vi "Write json to AIParam one test.vi"(10 "JSON Data In":string="AI  SET\n {\"GM1QN3_XQ01\":{\"instrument_gain\":10,\n                                    \"input_register_min\":6554,\n                                     \"input_register_max\":32767,\n                                     \"input_pv_max\":2.5},\n \"GM1QN4_XQ01\":{\"instrument_gain\":10,\n                                    \"input_register_min\":6554,\n                                     \"input_register_max\":32767,\n                                      \"input_pv_max\":4.99}\n}") -> (0 "error out":errorcluster)   [LabVIEW 2019]
uses:
  Database/ctl/Coninfo.ctl
  projects/Additivs/Regulators/PROG/GM1_201007/enums/KFM.ctl
  projects/Additivs/Regulators/PROG/GM1_201007/enums/AI.ctl
  projects/Graphetron_1/Heater/PROG/GM3_200601/enums/AI.ctl
  projects/Graphetron_1/Heater/PROG/GM3_200601/enums/KFM.ctl
  Transform/JSON to array.vi
  <vilib>/JDP Science/JSONtext/Find Multiple Items.vi
  <vilib>/JDP Science/JSONtext/String Subset.vi
  <vilib>/JDP Science/JSONtext/support/Strip Quotes and Unescape.vi
  <vilib>/JDP Science/JSONtext/Parsing/Parse Full Path or Item Name.vi
  <vilib>/JDP Science/JSONtext/Offset/Find Item Locations by Path.vi
  <vilib>/JDP Science/JSONtext/support/Unescape JSON string.vi
  <vilib>/JDP Science/JSONtext/Get Array Elements.vi
  projects/Graphetron_1/Heater/PROG/GM3_200601/enums/Param_gm3.lvlib
  Inputs.lvlib
  Database/PostgreSQL.lvlib
  projects/Additivs/Regulators/PROG/GM1_201007/enums/Param_h0gm1.lvlib
panel:
  in  "Set":bool
  in  "password":string
  in  "stop":bool
  out "data value 3":dbl[][](array[numeric])
  out "Names":string[][](array[string])
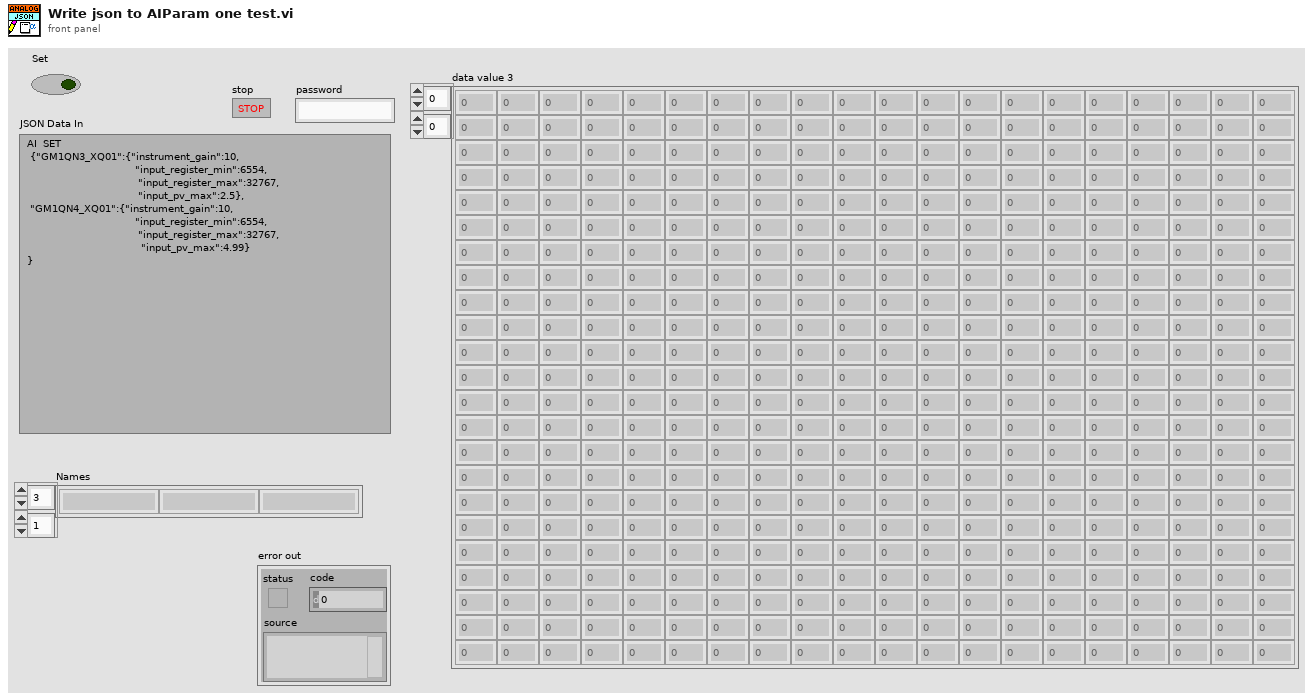
[diagram p1: front panel]
types:
  T1 = typedef "Param_h0gm1.lvlib/AI.ctl" = enum16{"GM1QN1_XQ01", "GM1QN2_XQ01", "GM1QN3_XQ01", "GM1QN4_XQ01", "GM1QN5_XQ01", "GM1QN6_XQ01", "GM1QN7_XQ01", "GM1QN8_XQ01", "GM1QN9_XQ01", "GM1QN10_XQ01", "GM1QN11_XQ01", "GM1QN12_XQ01", "GM1QN13_XQ01", "GM1QN14_XQ01", "GM1QN15_XQ01", "GM1QN16_XQ01", "GM1QN17_XQ01", "GM1QN18_XQ01", "GM1QN19_XQ01", "GM1QN20_XQ01", "GM1QN21_XQ01", "GM1QN22_XQ01", "GM1QN23_XQ01"}
  T2 = typedef "Param_h0gm1.lvlib/KFM.ctl" = enum16{"GM1JBA1_JA1", "GM1JBA1_JA2", "GM1JBA2_JA1", "GM1JBA2_JA2", "GM1JBA3_JA1"}
  T3 = typedef "PostgreSQL.lvlib/Coninfo.ctl" = cluster{"host":string, "port":string, "client_encoding":string, "dbname":string, "user":string, "password":string}
  T4 = enum16{"GM3KF1_A1", "EB2TB1_2TB1", "EB2TB2_2TB2", "EB2TB3_2TB3", "EB2TF1_A13", "EB2TF1_A131", "EB3TB1_3TB1", "EB3TB2_3TB2", "EB3TB3_3TB3", "GM2KF1_A1", "GM2KF1_A11", "GM2KF1_A12", "GM2KF1_A14", "GM2KF1_A15", "GM2KF1_A19", "GM2TF3_A117", "GM2TF3_A118", "GM3JBA1_A13", "GM3KF1_A11", "GM3KF1_A12", "GM3KF1_A15", "GM3KF1_A16", "GM3KF1_A17", "GM3KF1_A18", "GM3KF1_A19", "GM3TF1_A111", "GM3TF1_A112", "GM3TF1_A113", "GM3TF1_A114", "GM3TF1_A116", "GM3TF1_A117", "GM3TF1_A118", "GM3TF1_A14", "HXTF1_A11", "HXTF1_A14", "HXTF2_A15", "W2JBA1_A2", "W2JBA2_A2", "W2JBA3_A2", "W2JBA4_A2", "W2JBA5_A1"}
  T5 = typedef "Param_gm3.lvlib/KFM.ctl" = enum16{"GM3.KF1_A1", "EB2.TB.1_2TB1", "EB2.TB.2_2TB2", "EB2.TB.3_2TB3", "EB2.TF1_A13", "EB2.TF1_A131", "EB3.TB.1_3TB1", "EB3.TB.2_3TB2", "EB3.TB.3_3TB3", "GM2.KF1_A1", "GM2.KF1_A11", "GM2.KF1_A12", "GM2.KF1_A14", "GM2.KF1_A15", "GM2.KF1_A19", "GM2.TF3_A117", "GM2.TF3_A118", "GM3.JBA1_A13", "GM3.KF1_A11", "GM3.KF1_A12", "GM3.KF1_A15", "GM3.KF1_A16", "GM3.KF1_A17", "GM3.KF1_A18", "GM3.KF1_A19", "GM3.TF1_A111", "GM3.TF1_A112", "GM3.TF1_A113", "GM3.TF1_A114", "GM3.TF1_A116", "GM3.TF1_A117", "GM3.TF1_A118", "GM3.TF1_A14", "HX.TF1_A11", "HX.TF1_A14", "HX.TF2_A15", "W2.JBA1_A2", "W2.JBA2_A2", "W2.JBA3_A2", "W2.JBA4_A2", "W2.JBA5_A1"}
  T6 = enum16{"EB2BC11", "EB2BC12", "EB2BC21", "EB2BC22", "EB2BP1", "EB2BT1", "EB2BT2", "EB2BT3", "EB2BT4", "EB2BT5", "EB2QN1", "EB2QN2", "EB2TB1_BA1", "EB2TB1_BC1", "EB2TB1_BE1", "EB2TB1_BJ1", "EB2TB2_BA2", "EB2TB2_BC2", "EB2TB2_BE2", "EB2TB2_BJ2", "EB2TB3_BA3", "EB2TB3_BC3", "EB2TB3_BE3", "EB2TB3_BJ3", "EB2TB_BJ", "EB2_BC1", "EB2_BC2", "EB3BP1", "EB3BT11", "EB3BT12", "EB3BT21", "EB3BT22", "EB3BT31", "EB3BT32", "EB3QN1", "EB3QN2", "EB3TB1_BA1", "EB3TB1_BC1", "EB3TB1_BE1", "EB3TB1_BJ1", "EB3TB2_BA2", "EB3TB2_BC2", "EB3TB2_BE2", "EB3TB2_BJ2", "EB3TB3_BA3", "EB3TB3_BC3", "EB3TB3_BE3", "EB3TB3_BJ3", "EB3TB_BJ", "EB3_BC1", "EB3_BC2", "GM2EP1BT1", "GM2EP1BT10", "GM2EP1BT11", "GM2EP1BT2", "GM2EP1BT3", "GM2EP1BT4", "GM2EP1BT5", "GM2EP1BT6", "GM2EP1BT7", "GM2EP1BT8", "GM2EP1BT9", "GM31BP1", "GM31BP2", "GM31BW1", "GM31BW1_BQ01", "GM31BW1_BQ03", "GM31BW1_XZ01", "GM31BW2", "GM31BW2_BQ01", "GM31BW2_XZ01", "GM31QN1", "GM32BP1", "GM32QN1", "GM32QN2", "GM3HT1BC1", "GM3HT1BC2", "GM3HT1BT1", "GM3HT1BT2", "HW3BT1", "HW3BT2", "HW3BT3"}
  T7 = typedef "Param_gm3.lvlib/AI.ctl" = enum16{"EB2.BC11", "EB2.BC12", "EB2.BC21", "EB2.BC22", "EB2.BP1", "EB2.BT1", "EB2.BT2", "EB2.BT3", "EB2.BT4", "EB2.BT5", "EB2.QN1", "EB2.QN2", "EB2.TB.1_BA1", "EB2.TB.1_BC1", "EB2.TB.1_BE1", "EB2.TB.1_BJ1", "EB2.TB.2_BA2", "EB2.TB.2_BC2", "EB2.TB.2_BE2", "EB2.TB.2_BJ2", "EB2.TB.3_BA3", "EB2.TB.3_BC3", "EB2.TB.3_BE3", "EB2.TB.3_BJ3", "EB2.TB_BJ", "EB2_BC1", "EB2_BC2", "EB3.BP1", "EB3.BT11", "EB3.BT12", "EB3.BT21", "EB3.BT22", "EB3.BT31", "EB3.BT32", "EB3.QN1", "EB3.QN2", "EB3.TB.1_BA1", "EB3.TB.1_BC1", "EB3.TB.1_BE1", "EB3.TB.1_BJ1", "EB3.TB.2_BA2", "EB3.TB.2_BC2", "EB3.TB.2_BE2", "EB3.TB.2_BJ2", "EB3.TB.3_BA3", "EB3.TB.3_BC3", "EB3.TB.3_BE3", "EB3.TB.3_BJ3", "EB3.TB_BJ", "EB3_BC1", "EB3_BC2", "GM2.EP1.BT1", "GM2.EP1.BT10", "GM2.EP1.BT11", "GM2.EP1.BT2", "GM2.EP1.BT3", "GM2.EP1.BT4", "GM2.EP1.BT5", "GM2.EP1.BT6", "GM2.EP1.BT7", "GM2.EP1.BT8", "GM2.EP1.BT9", "GM3.1.BP1", "GM3.1.BP2", "GM3.1.BW1", "GM3.1.BW1_BQ01", "GM3.1.BW1_BQ03", "GM3.1.BW1_XZ01", "GM3.1.BW2", "GM3.1.BW2_BQ01", "GM3.1.BW2_XZ01", "GM3.1.QN1", "GM3.2.BP1", "GM3.2.QN1", "GM3.2.QN2", "GM3.HT1.BC1", "GM3.HT1.BC2", "GM3.HT1.BT1", "GM3.HT1.BT2", "HW3.BT1", "HW3.BT2", "HW3.BT3"}
  T8 = typedef "Inputs.lvlib/AI.ctl" = cluster{"AI_defs":T9, "modified":refnum<data-value>, "AIP":refnum<data-value>, "AINames":refnum<data-value>}
  T9 = typedef "Inputs.lvlib/AI short.ctl" = cluster{"AI":dbl[], "AIState":T10[], "AIALRState":errorcluster[]}
  T10 = typedef "Inputs.lvlib/Parameter State.ctl" = cluster{"code":i32, "visible":bool, "color":u32, "source":string}
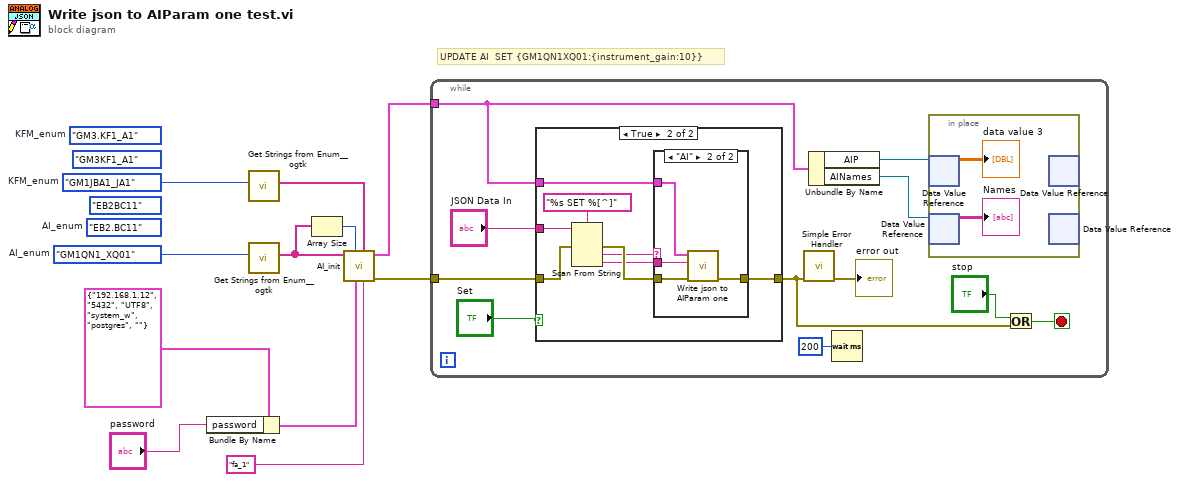
[diagram p0: block diagram]
diagram:
  w2 = AI."GM1QN1_XQ01"  # AI_enum
  w3 = KFM."GM1JBA1_JA1"  # KFM_enum
  (unwired) T4."GM3KF1_A1" ("KFM_enum")
  (unwired) KFM."GM3.KF1_A1"  # KFM_enum
  (unwired) T6."EB2BC11" ("AI_enum")
  (unwired) AI."EB2.BC11"  # AI_enum
  # "UPDATE AI  SET {GM1QN1XQ01:{instrument_gain:10}}"
  n1 = Bundle By Name(cluster=T3 {"host"="192.168.1.12", "port"="5432", "client_encoding"="UTF8", "dbname"="system_w", "user"="postgres", "password"=""} ("conninfo"), "password"="password") -> (w4:T3)
  n2 = call <userlib>:"Get Strings from Enum__ogtk.vi"("Enum"=w3) -> ("Enum Strings"=w8:string[])  [unwired: 7 in, 3 out]
  n3 = call <userlib>:"Get Strings from Enum__ogtk.vi"("Enum"=w2) -> ("Enum Strings"=w9:string[])  [unwired: 7 in, 3 out]
  n4 = Array Size(array=w9) -> (size(s)=w11:i32)
  n5 = call "AI_init.vi"("AIParamTable"="fa_1", "KFM"=w8, "conninfo"=w4, "N_param"=w11, "AIParameters"=w9) -> ("error"=w7:errorcluster, "AI out"=w1:T8)  [unwired: 5 in]
  n6 = while {
    tunnel: w7 -> [w22]
    tunnel: w1 -> [w17]
    stop <- w12 stop-if-true
    n7 = case shown="True" "Set" {
      tunnel: w22 -> [w25 w29]
      tunnel: [w25 w28] -> w13
      tunnel: "JSON Data In" -> [_ w27]
      tunnel: w17 -> [_ w26]
      frame False {
      }
      frame True {
        n8 = Scan From String(format string="%s SET %[^]", input string=w27, error in=w29) -> (error out=w32:errorcluster, output 1=w31:string, output 2=w30:string)  [unwired: 3 in, 2 out]
        n9 = case shown="\"AI\"" w31 {
          tunnel: w32 -> [w34 w37]
          tunnel: w30 -> [_ w38]
          tunnel: [w34 w36] -> w28
          tunnel: w26 -> [_ w35]
          frame "False", Default {
          }
          frame "AI" {
            n10 = call "Write json to AIParam one.vi"("error in (no error)"=w37, "JSON Data In"=w38, "AI in"=w35) -> ("error out"=w36:errorcluster)  [unwired: 7 in, 1 out]
          }
        }
      }
    }
    n11 = call <vilib>:"Simple Error Handler.vi"("error in (no error)"=w13) -> ("error out"=→"error out":errorcluster)  [unwired: 4 in, 4 out]
    n12 = Unbundle By Name(w17) -> ("AIP"=w16:refnum<data-value>, "AINames"=w15:refnum<data-value>)
    n13 = Wait (ms)(milliseconds to wait=u32 200) -> ()  [unwired: 1 out]
    n14 = in-place {
      n15 = in-place-dvr #1(w16) -> (→"data value 3":dbl[][])  [unwired: 1 out]
      n16 = in-place-dvr #2(w15) -> (→"Names":string[][])  [unwired: 1 out]
      n17 = in-place-dvr #1() -> ()  [unwired: 1 in, 2 out]
      n18 = in-place-dvr #2() -> ()  [unwired: 1 in, 2 out]
    }
    n19 = Or(x="stop", y=w13) -> (x .or. y?=w12:bool)
  }
